vi "Run List.vi"(8 "error in":errorcluster, 10 "Numeric":i32, 11 "VISA resource name":refnum<visa-resource-name>) -> (0 "error out":errorcluster, 3 "VISA resource name out":refnum<visa-resource-name>)   [LabVIEW 2022 SP3]
uses:
  <instrlib>/BK Precision 911X Series/BK Precision 911X Series.lvlib
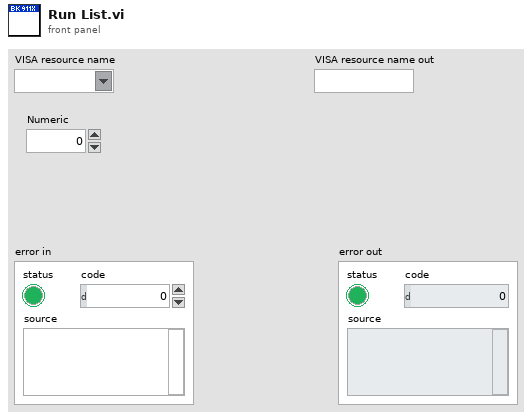
[diagram p1: front panel]
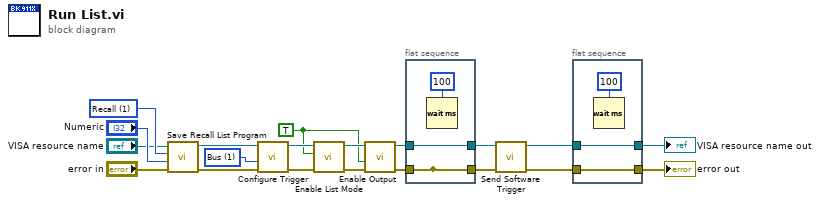
[diagram p0: block diagram]
diagram:
  w6 = 1 items=["Manual", "Bus"] ("Trigger Source (0:Manual)")
  w16 = u16 1 items=["Save", "Recall"] ("Save Recall List File (0:Save)")
  w1 = TRUE
  n1 = call <instrlib>:"Save Recall List Program.vi"("error in (no error)"="error in", "List Number (1)"="Numeric", "Save Recall List File (0:Save)"=w16, "VISA resource name"="VISA resource name") -> ("error out"=w7:errorcluster, "VISA resource name out"=w10:refnum<visa-resource-name>)  [unwired: 6 in]
  n2 = call <instrlib>:"Configure Trigger.vi"("error in (no error)"=w7, "Trigger Source (0:Manual)"=w6, "VISA resource name"=w10) -> ("error out"=w8:errorcluster, "VISA resource name out"=w9:refnum<visa-resource-name>)  [unwired: 7 in]
  n3 = call <instrlib>:"Enable List Mode.vi"("error in (no error)"=w8, "Enable List Mode (F: False)"=w1, "VISA resource name"=w9) -> ("error out"=w19:errorcluster, "VISA resource name out"=w20:refnum<visa-resource-name>)  [unwired: 7 in]
  n4 = call <instrlib>:"Enable Output.vi"("error in (no error)"=w19, "Enable Output (F: False)"=w1, "VISA resource name"=w20) -> ("error out"=w18:errorcluster, "VISA resource name out"=w17:refnum<visa-resource-name>)  [unwired: 7 in]
  n5 = flat-sequence {
    tunnel: w18 -> [w21]
    tunnel: [w21] -> _
    tunnel: [w22] -> w12
    tunnel: w17 -> [w22]
    tunnel: [w21] -> w11
    frame #0 {
      n6 = Wait (ms)(milliseconds to wait=u32 100) -> ()  [unwired: 1 out]
    }
  }
  n7 = call <instrlib>:"Send Software Trigger.vi"("error in (no error)"=w11, "VISA resource name"=w12) -> ("error out"=w3:errorcluster, "VISA resource name out"=w5:refnum<visa-resource-name>)  [unwired: 8 in]
  n8 = flat-sequence {
    tunnel: w3 -> [w24]
    tunnel: [w25] -> w4
    tunnel: w5 -> [w25]
    tunnel: [w24] -> w2
    frame #0 {
      n9 = Wait (ms)(milliseconds to wait=u32 100) -> ()  [unwired: 1 out]
    }
  }
  "VISA resource name out" <- w4
  "error out" <- w2
